vi "Muxed_Acquisition_1channel.vi"() -> ()   [LabVIEW 2014]
uses:
  <vilib>/rvi/Emulation/niFpgaGetClockAttributes.vi
  <vilib>/rvi/Emulation/niFpgaSctlEmulationGetInTimedLoop.vi
  <vilib>/rvi/Emulation/niFpgaEmulationReportErrorSimple.vi
  <vilib>/rvi/eio/common/nirviEmuTemplateMethod_errors.vi
  <vilib>/rvi/interface/RandomDataEmulation/niFpgaRandomDataHandleErrors.vi
  <vilib>/rvi/Emulation/niFpgaCriticalErrorInLSC.vi
  <vilib>/eio/EIONode/EIONode.xnode
  <vilib>/rvi/DataTransferAndStorage/Container/XNode/niFpgaContainer.xnode
  <vilib>/rvi/interface/RandomDataEmulation/nirviRandomDataFpgaReadWriteTemplate.vi
panel:
  out "Read Value":i16
  out "FIFO timeout":bool
  in  "Numeric":i16
  in  "Sampling(Ticks)":u32 caption="Count(Ticks)"
  out "Acquisition\nTimeout":bool
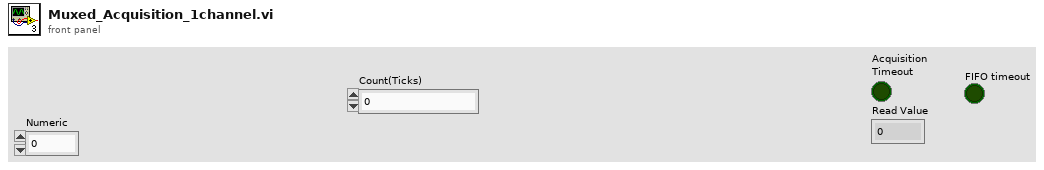
[diagram p1: front panel]
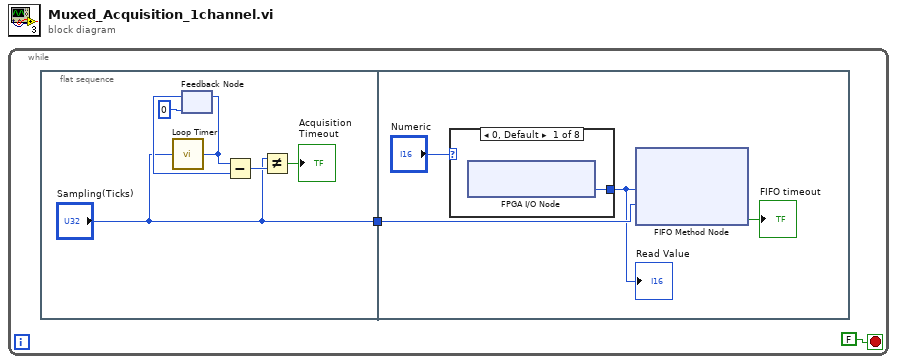
[diagram p0: block diagram]
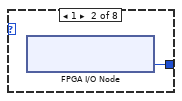
[diagram p2: hidden frame]
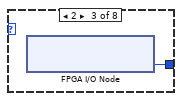
[diagram p3: hidden frame]
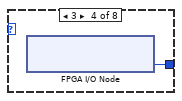
[diagram p4: hidden frame]
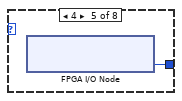
[diagram p5: hidden frame]
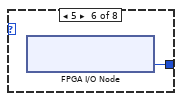
[diagram p6: hidden frame]
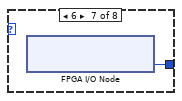
[diagram p7: hidden frame]
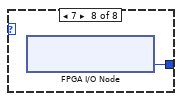
[diagram p8: hidden frame]
diagram:
  n1 = while {
    stop <- FALSE stop-if-true
    n2 = flat-sequence {
      tunnel: ["Sampling(Ticks)"] -> w1
      tunnel: w1 -> [w12]
      frame #0 {
        n3 = call "Loop Timer"("Count(Ticks)"="Sampling(Ticks)") -> ("Tick Count(Ticks)"=w7:u32)
        n4 = feedback-in #1(w7) -> ()
        n5 = feedback #1(u32 0 ("Tick Count(Ticks)")) -> (w6:u32)
        n6 = Subtract(x=w7, y=w6) -> (x-y=w5:u32)
        n7 = Not Equal?(x="Sampling(Ticks)", y=w5) -> (x != y?=→"Acquisition\nTimeout":bool)
      }
      frame #1 {
        n8 = case shown="0, Default" "Numeric" {
          tunnel: [w13 w14 w15 w16 w17 w18 w19 w20] -> w10
          frame 0, Default {
            n9 = xnode "FPGA I/O Node"() -> ("Connector0/AI0"=w13:i16)  [unwired: 1 in, 1 out]
          }
          frame 1 {
            n10 = xnode "FPGA I/O Node"() -> ("Connector0/AI1"=w14:i16)  [unwired: 1 in, 1 out]
          }
          frame 2 {
            n11 = xnode "FPGA I/O Node"() -> ("Connector0/AI2"=w15:i16)  [unwired: 1 in, 1 out]
          }
          frame 3 {
            n12 = xnode "FPGA I/O Node"() -> ("Connector0/AI3"=w16:i16)  [unwired: 1 in, 1 out]
          }
          frame 4 {
            n13 = xnode "FPGA I/O Node"() -> ("Connector0/AI4"=w17:i16)  [unwired: 1 in, 1 out]
          }
          frame 5 {
            n14 = xnode "FPGA I/O Node"() -> ("Connector0/AI5"=w18:i16)  [unwired: 1 in, 1 out]
          }
          frame 6 {
            n15 = xnode "FPGA I/O Node"() -> ("Connector0/AI6"=w19:i16)  [unwired: 1 in, 1 out]
          }
          frame 7 {
            n16 = xnode "FPGA I/O Node"() -> ("Connector0/AI7"=w20:i16)  [unwired: 1 in, 1 out]
          }
        }
        "Read Value" <- w10
        n17 = xnode ("FIFO Method Node")("Element"=w10, "Timeout"=w12) -> ("Timed Out?"=→"FIFO timeout":bool)  [unwired: 1 in, 1 out]
      }
    }
  }
